vi "lectura_simultanea_case_v2.vi"() -> ()   [LabVIEW 2020]
uses:
  <vilib>/BLE/type_def/connection_status_bundle.ctl
  <vilib>/BLE/type_def/address_type.ctl
  <vilib>/Utility/file.llb/Read Delimited Spreadsheet (string).vi
panel:
  out "Batería":u8(slide) scale=0.0..100.0
  in  "Tab Control":T1(tab)
  in  "Modo escritura":bool
  out "Temperatura":string caption="Result"
  out "Temp":dbl
  out "Presión":dbl
  out "Humedad":string caption="Result"
  in  "Leer color":bool
  out "Color":u32(colorbox)
  out "eCO2 ppm":u8
  out "TVOC ppb":u8
  in  "Intervalo Humedad":u16
  in  "Intervalo Temperatura":u16
  in  "Intervalo Presion":u16
  in  "Intervalo Color":u16
  in  "Modo Aire":u8
  in  "Intensidad Rojo":u8
  in  "Intensidad Verde":u8
  in  "Intensidad Azul":u8
  in  "Leer Boton":bool
  in  "Modo escritura":bool
  in  "Color (constant)":u32(colorbox)
  in  "Modo":u8
  in  "Intensidad (One Shot)":u8
  in  "Intensidad (breathe)":u8
  in  "Color (Breathe)":u8
  in  "Color (One Shot)":u8
  in  "Delay (breathe)":u16
  out "Botón pulsado":bool
  in  "Leer pasos":bool
  in  "Leer Orientacion":bool
  out "w 4":dbl
  out "x 4":dbl
  out "y 4":dbl
  out "z 4":dbl
  in  "Leer Quaternion":bool
  out "Orientacion":u8
  out "Tiempo":u32
  out "Pasos":u32
  in  "Leer gravedad":bool
  out "z":dbl
  out "y":dbl
  out "x":dbl
  in  "Sample":u8
  in  "Enviar sample":bool
  out "UIDS":string[][](array[string])
  in  "stop":bool
  out "MAC Address":string
  out "Connected":bool
  in  "Address Type":T2=1 items=["Public", "Random"]
  out "Handle table":string[][](array[string])
  out "Connection Status":T3={"MAC Address"="", "cnx handle"=0, "cnx flags"=0, "Address Type"=125, "Connection Interval (ms)"=125, "Timeout(ms)"=125, "Latency"=0, "bonding handle"=0} {"Address Type" items=["Public", "Random"]}
  in  "COM Bluegiga in":refnum<visa-resource-name>="COM13"
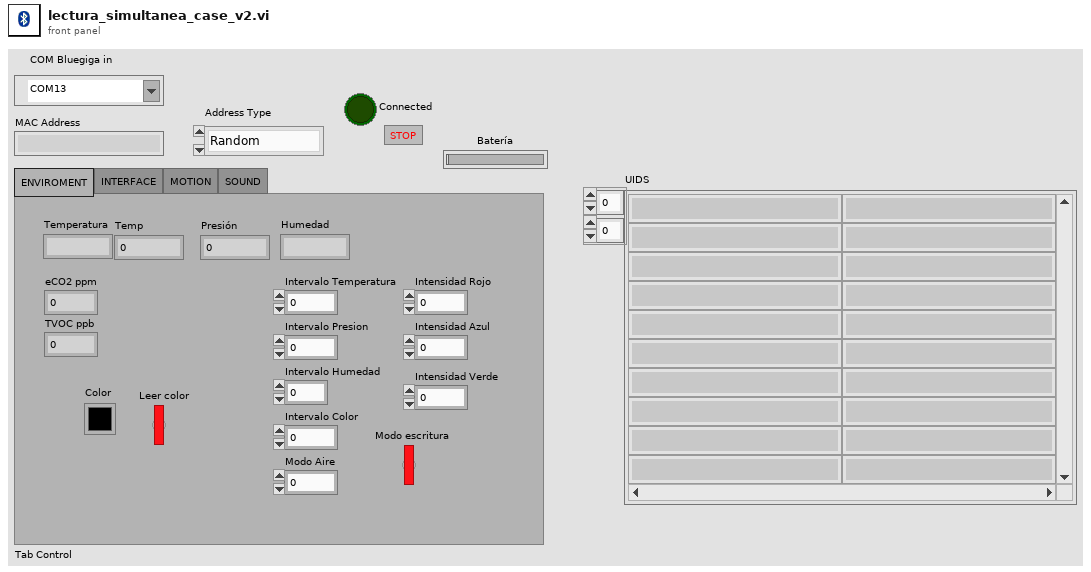
[diagram p1: front panel]
types:
  T1 = enum32{"ENVIROMENT", "INTERFACE", "MOTION", "SOUND"}
  T2 = typedef "address_type.ctl" = u8
  T3 = typedef "connection_status_bundle.ctl" = cluster{"MAC Address":string, "cnx handle":u8, "cnx flags":u8, "Address Type":T2, "Connection Interval (ms)":u16, "Timeout(ms)":u16, "Latency":u16, "bonding handle":u8}
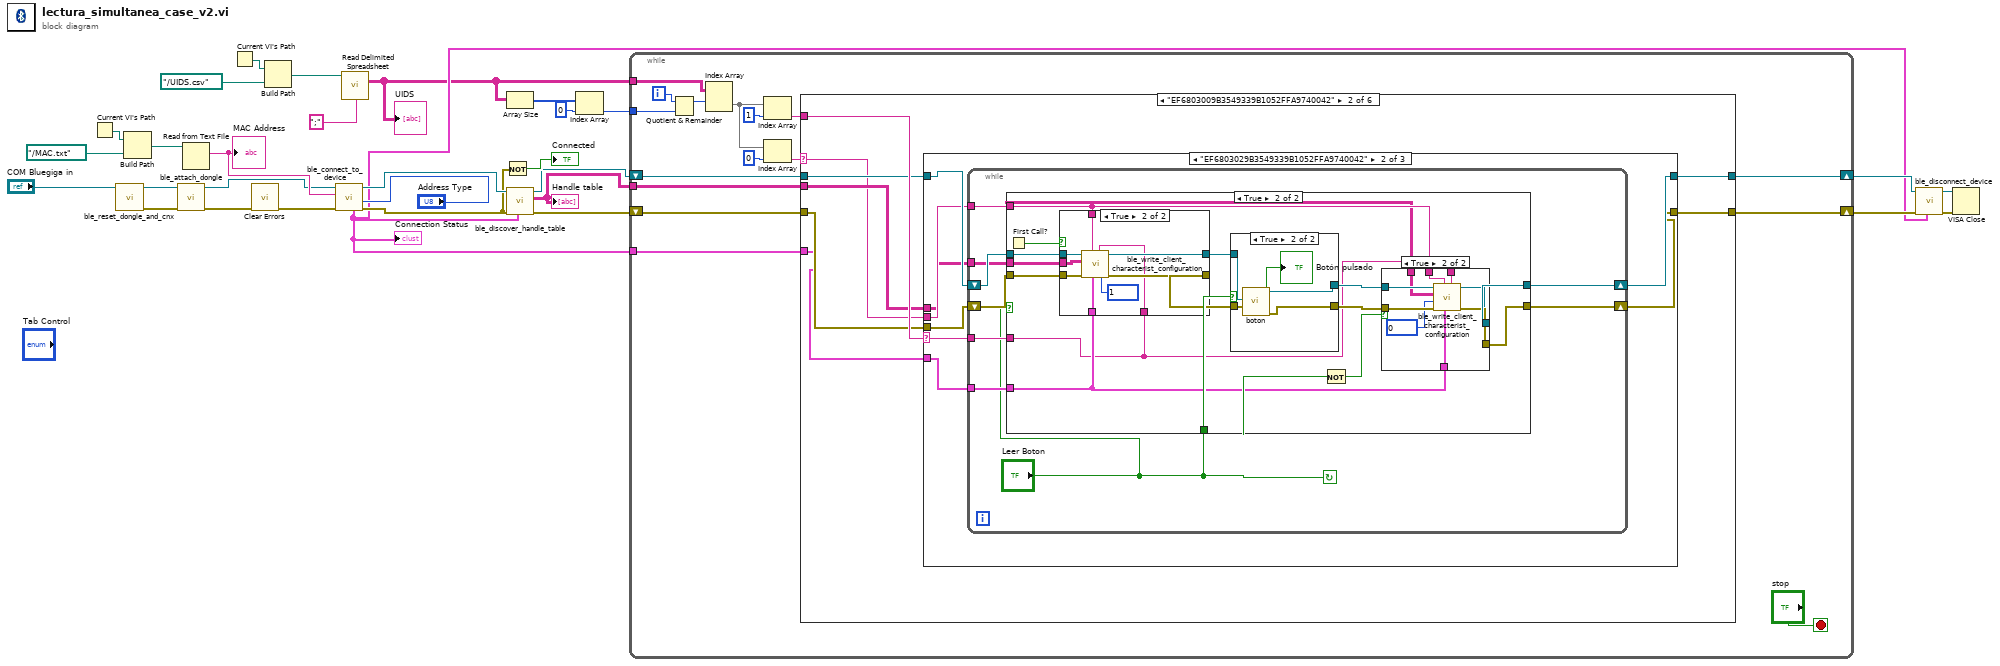
[diagram p0: block diagram]
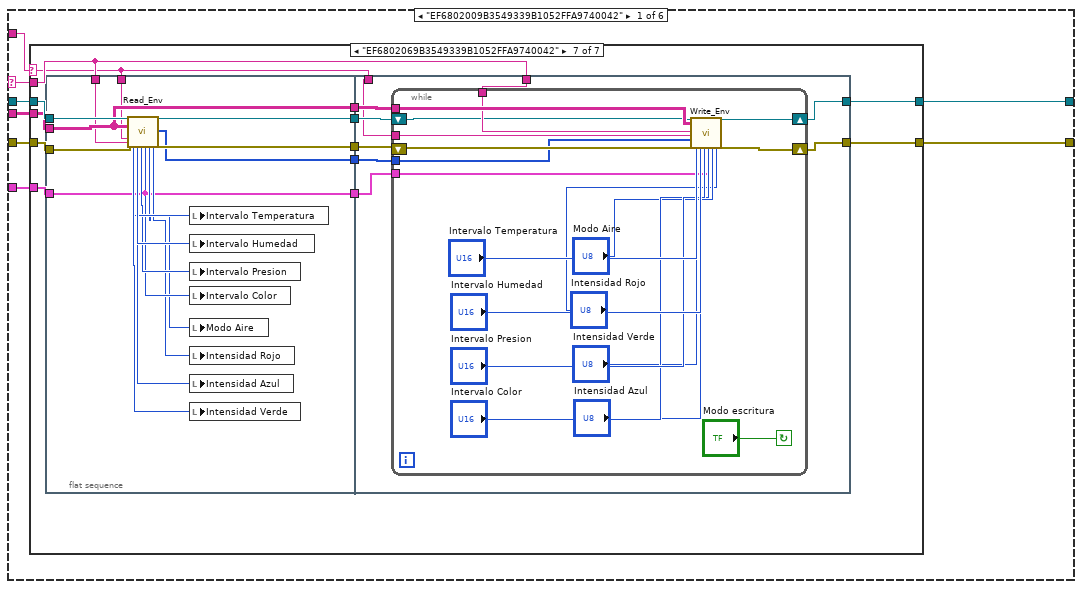
[diagram p2: hidden frame]
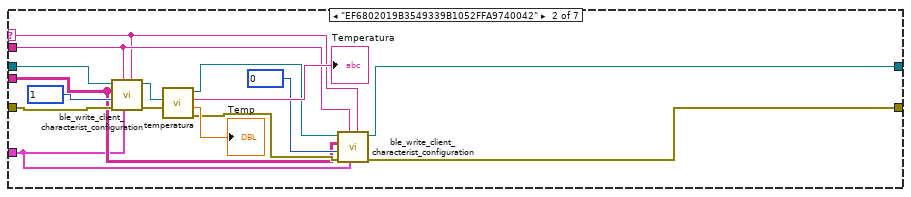
[diagram p4: hidden frame]
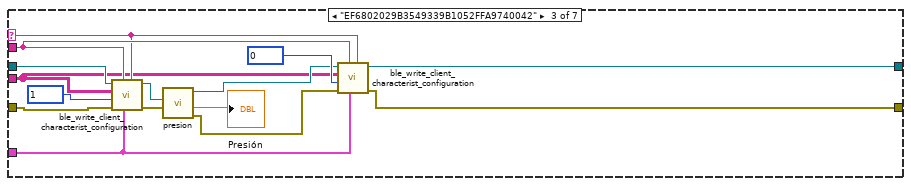
[diagram p5: hidden frame]
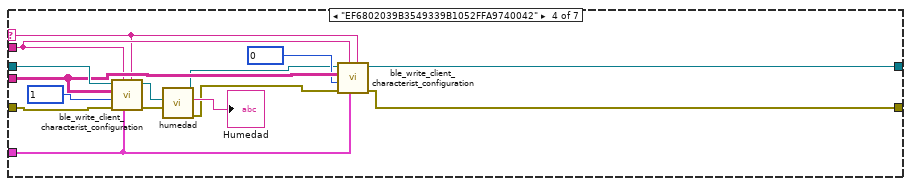
[diagram p6: hidden frame]
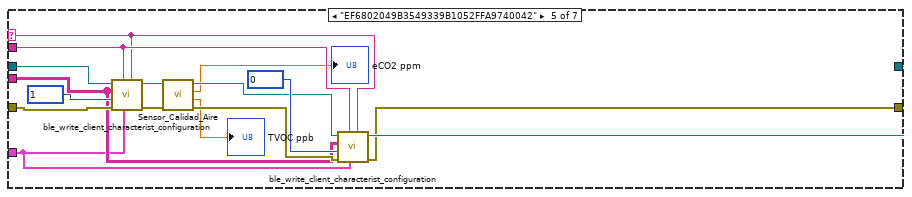
[diagram p7: hidden frame]
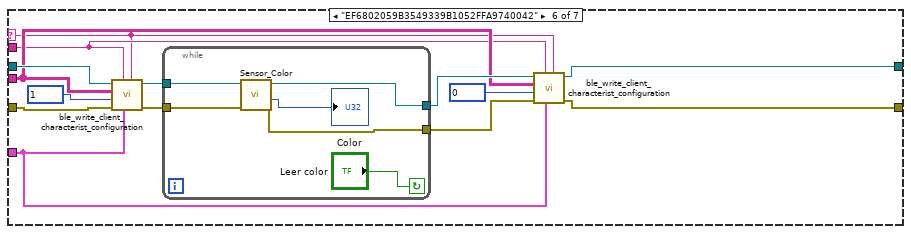
[diagram p8: hidden frame]
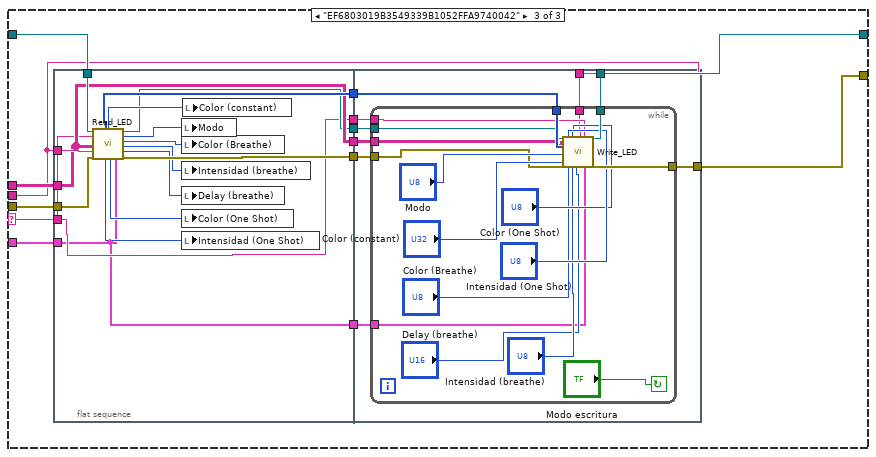
[diagram p14: hidden frame]
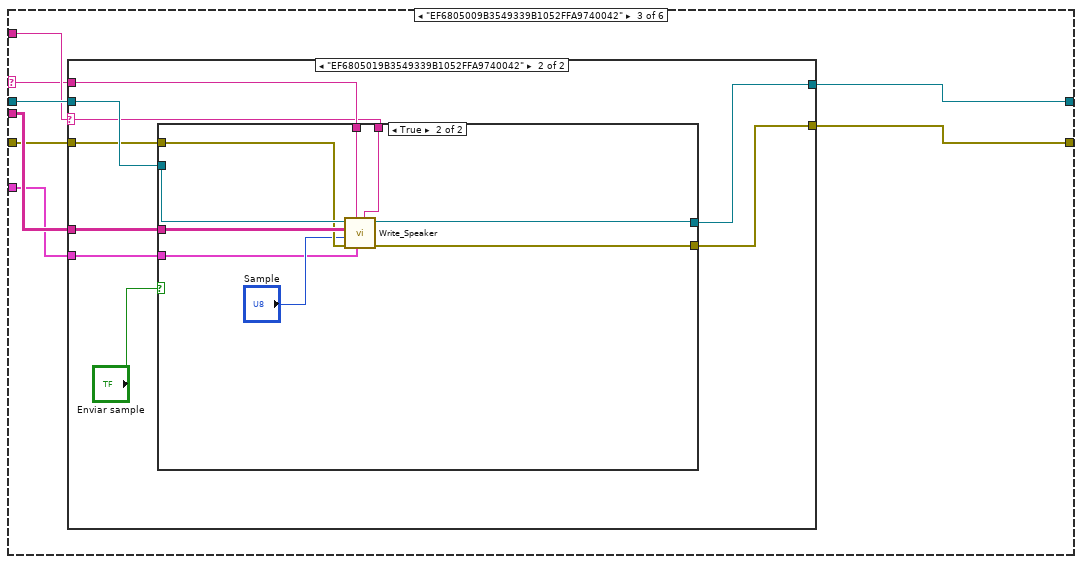
[diagram p15: hidden frame]
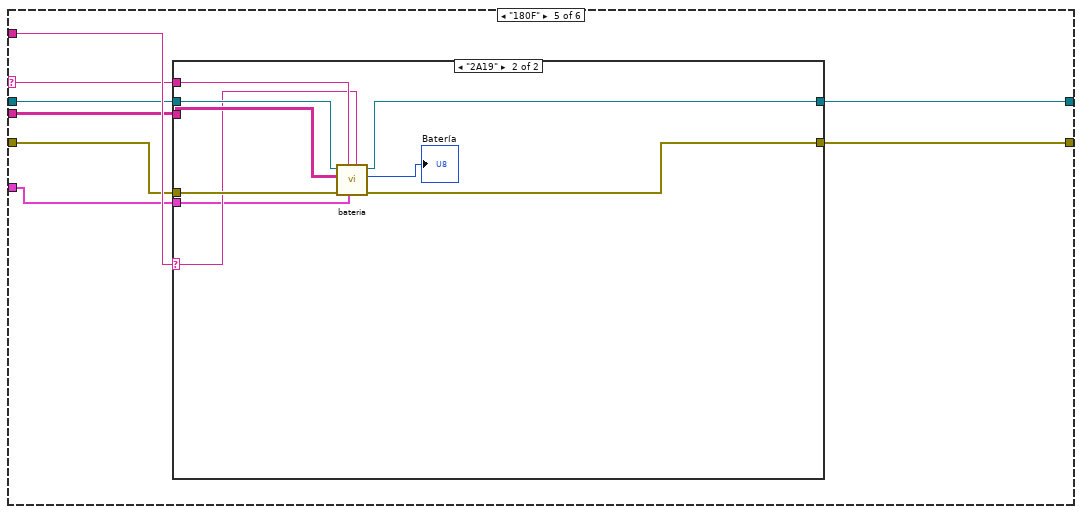
[diagram p19: hidden frame]
diagram:
  n1 = Current VI's Path() -> (path=w18:path)
  n2 = call <vilib>:"ble_reset_dongle_and_cnx.vi"("COM Bluegiga in"="COM Bluegiga in") -> ("error out"=w28:errorcluster, "COM Bluegiga out"=w26:refnum<visa-resource-name>)  [unwired: 9 in]
  n3 = Build Path(base path=w18, name or relative path=path "../MAC.txt") -> (appended path=w19:path)
  n4 = call <vilib>:"ble_attach_dongle.vi"("error in (no error)"=w28, "COM Bluegiga in"=w26) -> ("error out"=w16:errorcluster, "COM Bluegiga out"=w17:refnum<visa-resource-name>)  [unwired: 8 in]
  n5 = Read from Text File(file (use dialog)=w19) -> (text=w21:string)  [unwired: 3 in, 3 out]
  "MAC Address" <- w21
  n6 = Current VI's Path() -> (path=w7:path)
  n7 = call <vilib>:"Clear Errors.vi"("error in (no error)"=w16) -> ("error out"=w23:errorcluster)  [unwired: 5 in, 1 out]
  n8 = Build Path(base path=w7, name or relative path=path "../UIDS.csv") -> (appended path=w6:path)
  n9 = call <vilib>:"ble_connect_to_device.vi"("Address Type"="Address Type", "error in (no error)"=w23, "MAC Address"=w21, "COM Bluegiga in"=w17) -> ("error out"=w24:errorcluster, "COM Bluegiga out"=w25:refnum<visa-resource-name>, "Connection Status"=w12:T3)  [unwired: 5 in]
  "Connection Status" <- w12
  n10 = call-poly <vilib>:"Read Delimited Spreadsheet.vi"("file path (dialog if empty)"=w6, "delimiter (\\t)"=";" ("delimiter (\\t)")) -> ("all rows"=w2:string[][])  [unwired: 8 in, 5 out]
  "UIDS" <- w2
  n11 = Not(x=w24) -> (.not. x?=→"Connected":bool)
  n12 = Array Size(array=w2) -> (size(s)=w4:i32[])
  n13 = call <vilib>:"ble_discover_handle_table.vi"("Connection Status"=w12, "error in (no error)"=w24, "COM Bluegiga in"=w25) -> ("error out"=w10:errorcluster, "Handle table"=w11:string[][], "COM Bluegiga out"=w9:refnum<visa-resource-name>)  [unwired: 6 in]
  "Handle table" <- w11
  n14 = Index Array(array=w4, index=0) -> (element=w3:i32)
  n15 = while {
    tunnel: w2 -> [w32]
    shift-right: [w43] -> w13
    shift-left: w10 -> [w46]
    shift-right: [w44] -> w14
    shift-left: w9 -> [w45]
    tunnel: w12 -> [w42]
    tunnel: w11 -> [w41]
    tunnel: w3 -> [w31]
    i -> [w40]
    stop <- "stop" stop-if-true
    n16 = Quotient & Remainder(x=w40, y=w31) -> (x-y*floor(x/y)=w38:i32)  [unwired: 1 out]
    n17 = Index Array(array=w32, index (row)=w38) -> (element=w37:string[])  [unwired: 1 in]
    n18 = Index Array(array=w37, index=1) -> (element=w33:string)
    n19 = Index Array(array=w37, index=0) -> (element=w34:string)
    n20 = case shown="\"EF6803009B3549339B1052FFA9740042\"" w34 {
      selector: w34 -> [w53 w200 w326 _ w360 w376]
      tunnel: w46 -> [w50 w199 w330 w355 w361 w381]
      tunnel: w45 -> [w52 w202 w332 w356 w363 w382]
      tunnel: [w48 w197 w327 w356 w358 w379] -> w44
      tunnel: [w47 w196 w328 w355 w357 w378] -> w43
      tunnel: w42 -> [w49 w198 w325 _ w359 w380]
      tunnel: w41 -> [w51 w201 w331 _ w362 w377]
      tunnel: w33 -> [w54 w203 w329 _ w364 w383]
      frame "EF6802009B3549339B1052FFA9740042" {
        n21 = case shown="\"EF6802069B3549339B1052FFA9740042\"" w54 {
          selector: w54 -> [_ w57 w79 w97 w106 w120 w145]
          tunnel: w53 -> [_ w58 w80 w98 w107 w121 w146]
          tunnel: w52 -> [w56 w64 w78 w101 w112 w124 w149]
          tunnel: w51 -> [_ w62 w76 w99 w108 w122 w148]
          tunnel: w50 -> [w55 w63 w77 w100 w109 w123 w150]
          tunnel: w49 -> [_ w61 w83 w96 w103 w119 w141]
          tunnel: [w56 w59 w74 w95 w111 w126 w140] -> w48
          tunnel: [w55 w60 w73 w94 w110 w125 w139] -> w47
          frame Default {
          }
          frame "EF6802019B3549339B1052FFA9740042" {
            n22 = call <vilib>:"ble_write_client_characterist_configuration.vi"("Characteristic UUID"=w57, "Connection Status"=w61, "Service UUID"=w58, "error in (no error)"=w63, "Value(16bit)"=u16 1, "Handle table"=w62, "COM Bluegiga in"=w64) -> ("error out"=w70:errorcluster, "COM Bluegiga out"=w69:refnum<visa-resource-name>)  [unwired: 3 in]
            n23 = call "temperatura.vi"("error in (no error)"=w70, "COM Bluegiga in"=w69) -> ("error out"=w68:errorcluster, "Numeric"=→"Temp":dbl, "Text"=→"Temperatura":string, "COM Bluegiga out"=w67:refnum<visa-resource-name>)  [unwired: 6 in]
            n24 = call <vilib>:"ble_write_client_characterist_configuration.vi"("Characteristic UUID"=w57, "Connection Status"=w61, "Service UUID"=w58, "error in (no error)"=w68, "Value(16bit)"=u16 0, "Handle table"=w62, "COM Bluegiga in"=w67) -> ("error out"=w60:errorcluster, "COM Bluegiga out"=w59:refnum<visa-resource-name>)  [unwired: 3 in]
          }
          frame "EF6802029B3549339B1052FFA9740042" {
            n25 = call <vilib>:"ble_write_client_characterist_configuration.vi"("Characteristic UUID"=w79, "Connection Status"=w83, "Service UUID"=w80, "error in (no error)"=w77, "Value(16bit)"=u16 1, "Handle table"=w76, "COM Bluegiga in"=w78) -> ("error out"=w84:errorcluster, "COM Bluegiga out"=w85:refnum<visa-resource-name>)  [unwired: 3 in]
            n26 = call "presion.vi"("error in (no error)"=w84, "COM Bluegiga in"=w85) -> ("error out"=w82:errorcluster, "Presión"=→"Presión":dbl, "COM Bluegiga out"=w81:refnum<visa-resource-name>)  [unwired: 7 in]
            n27 = call <vilib>:"ble_write_client_characterist_configuration.vi"("Characteristic UUID"=w79, "Connection Status"=w83, "Service UUID"=w80, "error in (no error)"=w82, "Value(16bit)"=u16 0, "Handle table"=w76, "COM Bluegiga in"=w81) -> ("error out"=w73:errorcluster, "COM Bluegiga out"=w74:refnum<visa-resource-name>)  [unwired: 3 in]
          }
          frame "EF6802039B3549339B1052FFA9740042" {
            n28 = call <vilib>:"ble_write_client_characterist_configuration.vi"("Characteristic UUID"=w97, "Connection Status"=w96, "Service UUID"=w98, "error in (no error)"=w100, "Value(16bit)"=u16 1, "Handle table"=w99, "COM Bluegiga in"=w101) -> ("error out"=w90:errorcluster, "COM Bluegiga out"=w91:refnum<visa-resource-name>)  [unwired: 3 in]
            n29 = call "humedad.vi"("error in (no error)"=w90, "COM Bluegiga in"=w91) -> ("error out"=w88:errorcluster, "Text"=→"Humedad":string, "COM Bluegiga out"=w89:refnum<visa-resource-name>)  [unwired: 7 in]
            n30 = call <vilib>:"ble_write_client_characterist_configuration.vi"("Characteristic UUID"=w97, "Connection Status"=w96, "Service UUID"=w98, "error in (no error)"=w88, "Value(16bit)"=u16 0, "Handle table"=w99, "COM Bluegiga in"=w89) -> ("error out"=w94:errorcluster, "COM Bluegiga out"=w95:refnum<visa-resource-name>)  [unwired: 3 in]
          }
          frame "EF6802049B3549339B1052FFA9740042" {
            n31 = call <vilib>:"ble_write_client_characterist_configuration.vi"("Characteristic UUID"=w106, "Connection Status"=w103, "Service UUID"=w107, "error in (no error)"=w109, "Value(16bit)"=u16 1, "Handle table"=w108, "COM Bluegiga in"=w112) -> ("error out"=w114:errorcluster, "COM Bluegiga out"=w115:refnum<visa-resource-name>)  [unwired: 3 in]
            n32 = call "Sensor_Calidad_Aire.vi"("COM Bluegiga in"=w115, "error in (no error)"=w114) -> ("COM Bluegiga out"=w116:refnum<visa-resource-name>, "eCO2 ppm"=→"eCO2 ppm":dbl, "TVOC ppb"=→"TVOC ppb":dbl, "error out"=w113:errorcluster)  [unwired: 5 in]
            n33 = call <vilib>:"ble_write_client_characterist_configuration.vi"("Characteristic UUID"=w106, "Connection Status"=w103, "Service UUID"=w107, "error in (no error)"=w113, "Value(16bit)"=u16 0, "Handle table"=w108, "COM Bluegiga in"=w116) -> ("error out"=w110:errorcluster, "COM Bluegiga out"=w111:refnum<visa-resource-name>)  [unwired: 3 in]
          }
          frame "EF6802059B3549339B1052FFA9740042" {
            n34 = call <vilib>:"ble_write_client_characterist_configuration.vi"("Characteristic UUID"=w120, "Connection Status"=w119, "Service UUID"=w121, "error in (no error)"=w123, "Value(16bit)"=u16 1, "Handle table"=w122, "COM Bluegiga in"=w124) -> ("error out"=w129:errorcluster, "COM Bluegiga out"=w130:refnum<visa-resource-name>)  [unwired: 3 in]
            n35 = while {
              tunnel: w130 -> [w136]
              tunnel: w129 -> [w137]
              tunnel: [w135] -> w128
              tunnel: [w134] -> w127
              stop <- "Leer color" continue-if-true
              n36 = call "Sensor_Color.vi"("COM Bluegiga in"=w136, "error in (no error)"=w137) -> ("COM Bluegiga out"=w135:refnum<visa-resource-name>, "Color"=→"Color":u32, "error out"=w134:errorcluster)  [unwired: 5 in, 1 out]
            }
            n37 = call <vilib>:"ble_write_client_characterist_configuration.vi"("Characteristic UUID"=w120, "Connection Status"=w119, "Service UUID"=w121, "error in (no error)"=w127, "Value(16bit)"=u16 0, "Handle table"=w122, "COM Bluegiga in"=w128) -> ("error out"=w125:errorcluster, "COM Bluegiga out"=w126:refnum<visa-resource-name>)  [unwired: 3 in]
          }
          frame "EF6802069B3549339B1052FFA9740042" {
            n38 = flat-sequence {
              tunnel: [w160] -> w151
              tunnel: w150 -> [w159]
              tunnel: w149 -> [w158]
              tunnel: w148 -> [w157]
              tunnel: [w157] -> w147
              tunnel: w146 -> [w156]
              tunnel: w145 -> [w155]
              tunnel: [w154] -> w144
              tunnel: [w153] -> w143
              tunnel: [w152] -> w142
              tunnel: w141 -> [w152]
              tunnel: w151 -> [w177]
              tunnel: w147 -> [w176]
              tunnel: w146 -> [w175]
              tunnel: w145 -> [w174]
              tunnel: w144 -> [w173]
              tunnel: w143 -> [w172]
              tunnel: w142 -> [w171]
              tunnel: [w170] -> w140
              tunnel: [w169] -> w139
              frame #0 {
                n39 = call "Read_Env.vi"("COM Bluegiga in"=w158, "Handle table"=w157, "Characteristic UUID"=w155, "Service UUID"=w156, "error in (no error)"=w159, "Connection Status"=w152) -> ("Intervalo Temperatura"=w165:u16, "Intensidad Verde"=w167:u8, "Intervalo Humedad"=w168:u16, "Intensidad Azul"=w166:u8, "Intervalo Presion"=w164:u16, "Intervalo Color"=w163:u16, "Modo Aire"=w162:u8, "Intensidad Rojo"=w161:u8, "COM Bluegiga out"=w160:refnum<visa-resource-name>, "Registro Completo"=w153:u8[], "error out"=w154:errorcluster)  [unwired: 11 in]
                n40 = local write "Intervalo Temperatura"(w165) -> ()
                n41 = local write "Intervalo Humedad"(w168) -> ()
                n42 = local write "Intervalo Presion"(w164) -> ()
                n43 = local write "Intervalo Color"(w163) -> ()
                n44 = local write "Modo Aire"(w162) -> ()
                n45 = local write "Intensidad Rojo"(w161) -> ()
                n46 = local write "Intensidad Azul"(w166) -> ()
                n47 = local write "Intensidad Verde"(w167) -> ()
              }
              frame #1 {
                n48 = while {
                  shift-right: [w187] -> w170
                  shift-left: w177 -> [w180]
                  shift-right: [w186] -> w169
                  shift-left: w173 -> [w182]
                  tunnel: w176 -> [w185]
                  tunnel: w175 -> [w184]
                  tunnel: w174 -> [w183]
                  tunnel: w172 -> [w181]
                  tunnel: w171 -> [w179]
                  stop <- "Modo escritura" continue-if-true
                  n49 = call "Write_Env.vi"("COM Bluegiga in"=w180, "Handle table"=w185, "Service UUID"=w184, "Characteristic UUID"=w183, "Registro Completo"=w181, "error in (no error)"=w182, "Intervalo Temperatura"="Intervalo Temperatura", "Intensidad Verde"="Intensidad Verde", "Intervalo Humedad"="Intervalo Humedad", "Intensidad Azul"="Intensidad Azul", "Intervalo Presion"="Intervalo Presion", "Intervalo Color"="Intervalo Color", "Connection Status"=w179, "Modo Aire"="Modo Aire", "Intensidad Rojo"="Intensidad Rojo") -> ("COM Bluegiga out"=w187:refnum<visa-resource-name>, "error out"=w186:errorcluster)  [unwired: 11 in]
                }
              }
            }
          }
        }
      }
      frame "EF6803009B3549339B1052FFA9740042" {
        n50 = case shown="\"EF6803029B3549339B1052FFA9740042\"" w203 {
          selector: w203 -> [_ w210 w281]
          tunnel: w202 -> [w205 w213 w282]
          tunnel: w201 -> [_ w208 w280]
          tunnel: w200 -> [_ w209 w270]
          tunnel: w199 -> [w204 w212 w279]
          tunnel: w198 -> [_ w211 w278]
          tunnel: [w205 w207 w273] -> w197
          tunnel: [w204 w206 w272] -> w196
          frame "False", Default {
          }
          frame "EF6803029B3549339B1052FFA9740042" {
            n51 = while {
              shift-right: [w215] -> w206
              shift-left: w212 -> [w221]
              shift-right: [w216] -> w207
              shift-left: w213 -> [w222]
              tunnel: w211 -> [w220]
              tunnel: w210 -> [w219]
              tunnel: w209 -> [w218]
              tunnel: w208 -> [w217]
              stop <- "Leer Boton" continue-if-true
              n52 = case shown="True" "Leer Boton" {
                tunnel: "Leer Boton" -> [_ w236]
                tunnel: w222 -> [w224 w234]
                tunnel: w221 -> [w223 w233]
                tunnel: w220 -> [_ w230]
                tunnel: w219 -> [_ w229]
                tunnel: w218 -> [_ w228]
                tunnel: w217 -> [_ w227]
                tunnel: [w224 w226] -> w216
                tunnel: [w223 w225] -> w215
                frame False {
                }
                frame True {
                  n53 = First Call?() -> (First Call?: T/F=w237:bool)
                  n54 = case shown="True" w237 {
                    tunnel: w234 -> [w259 w267]
                    tunnel: w233 -> [w258 w266]
                    tunnel: [w259 w265] -> w232
                    tunnel: [w258 w264] -> w231
                    tunnel: w230 -> [_ w263]
                    tunnel: w229 -> [_ w262]
                    tunnel: w228 -> [_ w261]
                    tunnel: w227 -> [_ w260]
                    frame False {
                    }
                    frame True {
                      n55 = call <vilib>:"ble_write_client_characterist_configuration.vi"("Characteristic UUID"=w262, "Connection Status"=w263, "Service UUID"=w261, "error in (no error)"=w266, "Value(16bit)"=u16 1, "Handle table"=w260, "COM Bluegiga in"=w267) -> ("error out"=w264:errorcluster, "COM Bluegiga out"=w265:refnum<visa-resource-name>)  [unwired: 3 in]
                    }
                  }
                  n56 = case shown="True" w236 {
                    tunnel: [w240 w245] -> w239
                    tunnel: [w241 w244] -> w238
                    tunnel: w232 -> [w241 w243]
                    tunnel: w231 -> [w240 w242]
                    frame False {
                    }
                    frame True {
                      n57 = call "boton.vi"("error in (no error)"=w242, "COM Bluegiga in"=w243) -> ("error out"=w245:errorcluster, "Boolean output"=→"Botón pulsado":bool, "COM Bluegiga out"=w244:refnum<visa-resource-name>)  [unwired: 6 in, 1 out]
                    }
                  }
                  n58 = Not(x=w236) -> (.not. x?=w235:bool)
                  n59 = case shown="True" w235 {
                    tunnel: w239 -> [w247 w257]
                    tunnel: w238 -> [w248 w256]
                    tunnel: [w247 w255] -> w225
                    tunnel: [w248 w254] -> w226
                    tunnel: w230 -> [_ w252]
                    tunnel: w229 -> [_ w251]
                    tunnel: w228 -> [_ w250]
                    tunnel: w227 -> [_ w249]
                    frame False {
                    }
                    frame True {
                      n60 = call <vilib>:"ble_write_client_characterist_configuration.vi"("Characteristic UUID"=w251, "Connection Status"=w252, "Service UUID"=w250, "error in (no error)"=w257, "Value(16bit)"=u16 0, "Handle table"=w249, "COM Bluegiga in"=w256) -> ("error out"=w255:errorcluster, "COM Bluegiga out"=w254:refnum<visa-resource-name>)  [unwired: 3 in]
                    }
                  }
                }
              }
            }
          }
          frame "EF6803019B3549339B1052FFA9740042" {
            n61 = flat-sequence {
              tunnel: w282 -> [w298]
              tunnel: w281 -> [w284]
              tunnel: w280 -> [w286]
              tunnel: w270 -> [w297]
              tunnel: w279 -> [w296]
              tunnel: w278 -> [w283]
              tunnel: [w295] -> w277
              tunnel: [w287] -> w276
              tunnel: [w286] -> w275
              tunnel: [w285] -> w274
              tunnel: [w284] -> w271
              tunnel: [w283] -> w269
              tunnel: w277 -> [w304]
              tunnel: w276 -> [w307]
              tunnel: w275 -> [w306]
              tunnel: w274 -> [w305]
              tunnel: [w303] -> w273
              tunnel: [w302] -> w272
              tunnel: w271 -> [w301]
              tunnel: w270 -> [w300]
              tunnel: w269 -> [w299]
              frame #0 {
                n62 = call "Read_LED.vi"("COM Bluegiga in"=w298, "Characteristic UUID"=w284, "Handle table"=w286, "Service UUID"=w297, "error in (no error)"=w296, "Connection Status"=w283) -> ("Registro Completo"=w287:u8[], "Intensidad (One Shot)"=w289:u8, "Color (constant)"=w293:u32, "Color (One Shot)"=w288:u8, "COM Bluegiga out"=w285:refnum<visa-resource-name>, "Modo"=w294:u8, "Color (Breathe)"=w292:u8, "Intensidad (breathe)"=w290:u8, "Delay (breathe)"=w291:u16, "error out"=w295:errorcluster)  [unwired: 4 in]
                n63 = local write "Modo"(w294) -> ()
                n64 = local write "Color (Breathe)"(w292) -> ()
                n65 = local write "Intensidad (breathe)"(w290) -> ()
                n66 = local write "Delay (breathe)"(w291) -> ()
                n67 = local write "Color (One Shot)"(w288) -> ()
                n68 = local write "Intensidad (One Shot)"(w289) -> ()
                n69 = local write "Color (constant)"(w293) -> ()
              }
              frame #1 {
                n70 = while {
                  tunnel: w307 -> [w321]
                  tunnel: w306 -> [w320]
                  tunnel: w305 -> [w319]
                  tunnel: w304 -> [w318]
                  tunnel: [w317] -> w303
                  tunnel: [w316] -> w302
                  tunnel: w301 -> [w313]
                  tunnel: w300 -> [w312]
                  tunnel: w299 -> [w308]
                  stop <- "Modo escritura" continue-if-true
                  n71 = call "Write_LED.vi"("COM Bluegiga in"=w319, "Handle table"=w320, "Registro Completo"=w321, "Modo"="Modo", "Color (constant)"="Color (constant)", "error in (no error)"=w318, "Intensidad (One Shot)"="Intensidad (One Shot)", "Color (Breathe)"="Color (Breathe)", "Color (One Shot)"="Color (One Shot)", "Intensidad (breathe)"="Intensidad (breathe)", "Delay (breathe)"="Delay (breathe)", "Service UUID"=w312, "Characteristic UUID"=w313, "Connection Status"=w308) -> ("COM Bluegiga out"=w317:refnum<visa-resource-name>, "error out"=w316:errorcluster)  [unwired: 12 in]
                }
              }
            }
          }
        }
      }
      frame "EF6805009B3549339B1052FFA9740042" {
        n72 = case shown="\"EF6805019B3549339B1052FFA9740042\"" w329 {
          selector: w329 -> [_ w336]
          tunnel: [w334 w338] -> w327
          tunnel: [w333 w339] -> w328
          tunnel: w332 -> [w334 w342]
          tunnel: w331 -> [_ w341]
          tunnel: w330 -> [w333 w340]
          tunnel: w326 -> [_ w337]
          tunnel: w325 -> [_ w335]
          frame "False", Default {
          }
          frame "EF6805019B3549339B1052FFA9740042" {
            n73 = case shown="True" "Enviar sample" {
              tunnel: w342 -> [w345 w354]
              tunnel: w341 -> [_ w353]
              tunnel: w340 -> [w344 w352]
              tunnel: [w344 w350] -> w339
              tunnel: [w345 w349] -> w338
              tunnel: w337 -> [_ w348]
              tunnel: w336 -> [_ w346]
              tunnel: w335 -> [_ w347]
              frame False {
              }
              frame True {
                n74 = call "Write_Speaker.vi"("Characteristic UUID"=w346, "Connection Status"=w347, "Service UUID"=w348, "error in (no error)"=w352, "Sample"="Sample", "Handle table"=w353, "COM Bluegiga in"=w354) -> ("error out"=w350:errorcluster, "COM Bluegiga out"=w349:refnum<visa-resource-name>)  [unwired: 3 in]
              }
            }
          }
        }
      }
      frame Default {
      }
      frame "180F" {
        n75 = case shown="\"2A19\"" w364 {
          selector: w364 -> [_ w371]
          tunnel: w363 -> [w366 w375]
          tunnel: w362 -> [_ w374]
          tunnel: w361 -> [w365 w373]
          tunnel: w360 -> [_ w372]
          tunnel: w359 -> [_ w370]
          tunnel: [w366 w369] -> w358
          tunnel: [w365 w368] -> w357
          frame "False", Default {
          }
          frame "2A19" {
            n76 = call "bateria.vi"("Characteristic UUID"=w371, "Connection Status"=w370, "Service UUID"=w372, "error in (no error)"=w373, "Handle table"=w374, "COM Bluegiga in"=w375) -> ("error out"=w368:errorcluster, "Numeric"=→"Batería":u8, "COM Bluegiga out"=w369:refnum<visa-resource-name>)  [unwired: 2 in, 1 out]
          }
        }
      }
      frame "EF6804009B3549339B1052FFA9740042" {
        n77 = case shown="\"EF6804039B3549339B1052FFA9740042\"" w383 {
          selector: w383 -> [_ w388 w416 w439 w463]
          tunnel: w382 -> [w385 w394 w419 w443 w469]
          tunnel: w381 -> [w384 w393 w420 w442 w468]
          tunnel: w380 -> [_ w390 w414 w438 w462]
          tunnel: [w385 w392 w413 w436 w467] -> w379
          tunnel: [w384 w391 w412 w437 w466] -> w378
          tunnel: w377 -> [_ w387 w415 w441 w465]
          tunnel: w376 -> [_ w389 w417 w440 w464]
          frame Default {
          }
          frame "EF6804039B3549339B1052FFA9740042" {
            n78 = case shown="True" "Leer Orientacion" {
              tunnel: w394 -> [w396 w410]
              tunnel: w393 -> [w395 w409]
              tunnel: [w396 w408] -> w392
              tunnel: [w395 w407] -> w391
              tunnel: w390 -> [_ w406]
              tunnel: w389 -> [_ w405]
              tunnel: w388 -> [_ w404]
              tunnel: w387 -> [_ w403]
              frame False {
              }
              frame True {
                n79 = call <vilib>:"ble_write_client_characterist_configuration.vi"("Characteristic UUID"=w404, "Connection Status"=w406, "Service UUID"=w405, "error in (no error)"=w409, "Value(16bit)"=u16 1, "Handle table"=w403, "COM Bluegiga in"=w410) -> ("error out"=w401:errorcluster, "COM Bluegiga out"=w402:refnum<visa-resource-name>)  [unwired: 3 in]
                n80 = call "orientacion.vi"("COM Bluegiga in"=w402, "error in (no error)"=w401) -> ("Orientacion"=→"Orientacion":u8, "COM Bluegiga out"=w400:refnum<visa-resource-name>, "error out"=w399:errorcluster)  [unwired: 11 in, 4 out]
                n81 = call <vilib>:"ble_write_client_characterist_configuration.vi"("Characteristic UUID"=w404, "Connection Status"=w406, "Service UUID"=w405, "error in (no error)"=w399, "Value(16bit)"=u16 0, "Handle table"=w403, "COM Bluegiga in"=w400) -> ("error out"=w407:errorcluster, "COM Bluegiga out"=w408:refnum<visa-resource-name>)  [unwired: 3 in]
              }
            }
          }
          frame "EF6804049B3549339B1052FFA9740042" {
            n82 = call <vilib>:"ble_write_client_characterist_configuration.vi"("Characteristic UUID"=w416, "Connection Status"=w414, "Service UUID"=w417, "error in (no error)"=w420, "Value(16bit)"=u16 1, "Handle table"=w415, "COM Bluegiga in"=w419) -> ("error out"=w423:errorcluster, "COM Bluegiga out"=w422:refnum<visa-resource-name>)  [unwired: 3 in]
            n83 = while {
              shift-right: [w434] -> w425
              shift-left: w423 -> [w432]
              shift-right: [w433] -> w424
              shift-left: w422 -> [w431]
              stop <- "Leer Quaternion" continue-if-true
              n84 = call "quaternion.vi"("error in (no error)"=w432, "COM Bluegiga in"=w431) -> ("z"=→"z 4":dbl, "y"=→"y 4":dbl, "x"=→"x 4":dbl, "w"=→"w 4":dbl, "COM Bluegiga out"=w433:refnum<visa-resource-name>, "error out"=w434:errorcluster)  [unwired: 4 in]
            }
            n85 = call <vilib>:"ble_write_client_characterist_configuration.vi"("Characteristic UUID"=w416, "Connection Status"=w414, "Service UUID"=w417, "error in (no error)"=w425, "Value(16bit)"=u16 0, "Handle table"=w415, "COM Bluegiga in"=w424) -> ("error out"=w412:errorcluster, "COM Bluegiga out"=w413:refnum<visa-resource-name>)  [unwired: 3 in]
          }
          frame "EF6804059B3549339B1052FFA9740042" {
            n86 = case shown="True" "Leer pasos" {
              tunnel: w443 -> [w444 w460]
              tunnel: w442 -> [w445 w459]
              tunnel: w441 -> [_ w452]
              tunnel: w440 -> [_ w458]
              tunnel: w439 -> [_ w457]
              tunnel: w438 -> [_ w454]
              tunnel: [w445 w449] -> w437
              tunnel: [w444 w448] -> w436
              frame False {
              }
              frame True {
                n87 = call <vilib>:"ble_write_client_characterist_configuration.vi"("Characteristic UUID"=w457, "Connection Status"=w454, "Service UUID"=w458, "error in (no error)"=w459, "Value(16bit)"=u16 1, "Handle table"=w452, "COM Bluegiga in"=w460) -> ("error out"=w455:errorcluster, "COM Bluegiga out"=w456:refnum<visa-resource-name>)  [unwired: 3 in]
                n88 = call "steps.vi"("COM Bluegiga in"=w456, "error in (no error)"=w455) -> ("COM Bluegiga out"=w451:refnum<visa-resource-name>, "Tiempo"=→"Tiempo":u32, "Pasos"=→"Pasos":u32, "error out"=w450:errorcluster)  [unwired: 14 in]
                n89 = call <vilib>:"ble_write_client_characterist_configuration.vi"("error in (no error)"=w450, "Value(16bit)"=u16 0, "Handle table"=w452, "COM Bluegiga in"=w451) -> ("error out"=w449:errorcluster, "COM Bluegiga out"=w448:refnum<visa-resource-name>)  [unwired: 6 in]
              }
            }
          }
          frame "EF68040A9B3549339B1052FFA9740042" {
            n90 = call <vilib>:"ble_write_client_characterist_configuration.vi"("Characteristic UUID"=w463, "Connection Status"=w462, "Service UUID"=w464, "error in (no error)"=w468, "Value(16bit)"=u16 1, "Handle table"=w465, "COM Bluegiga in"=w469) -> ("error out"=w473:errorcluster, "COM Bluegiga out"=w472:refnum<visa-resource-name>)  [unwired: 3 in]
            n91 = while {
              shift-right: [w476] -> w475
              shift-left: w473 -> [w481]
              shift-right: [w477] -> w474
              shift-left: w472 -> [w482]
              stop <- "Leer gravedad" continue-if-true
              n92 = call "Read_Gravi.vi"("COM Bluegiga in"=w482, "error in (no error)"=w481) -> ("COM Bluegiga out"=w477:refnum<visa-resource-name>, "X"=→"x":ext, "Y"=→"y":ext, "Z"=→"z":ext, "error out"=w476:errorcluster)  [unwired: 9 in]
            }
            n93 = call <vilib>:"ble_write_client_characterist_configuration.vi"("Characteristic UUID"=w463, "Connection Status"=w462, "Service UUID"=w464, "error in (no error)"=w475, "Value(16bit)"=u16 0, "Handle table"=w465, "COM Bluegiga in"=w474) -> ("error out"=w466:errorcluster, "COM Bluegiga out"=w467:refnum<visa-resource-name>)  [unwired: 3 in]
          }
        }
      }
    }
  }
  n94 = call <vilib>:"ble_disconnect_device.vi"("Connection Status"=w12, "error in (no error)"=w13, "COM Bluegiga in"=w14) -> ("error out"=w29:errorcluster, "COM Bluegiga out"=w30:refnum<visa-resource-name>)  [unwired: 7 in]
  n95 = VISA Close(VISA resource name=w30, error in (no error)=w29) -> ()  [unwired: 1 out]
